vi "Subvi_Online_SVM_SWLDA_1세부통합.vi"(0 "rate":dbl=500.0 caption="Rate" format="%0.2f", 1 "Value":T1, 2 "Matrix":T1, 3 "in":T1, 5 "samples per channel":i32=25, 9 "Brain_data_source":dbl[][](array[numeric]) caption="EEG_Raw_Data" format="%0.3f", 11 "Target_Flash_Order":i64[][](array[numeric])) -> (4 "output-0~8":i32, 6 "decision":dbl[](array[numeric]), 8 "ERP_발생여부":bool, 10 "SWLDA":dbl[](array[numeric]), 13 "EPR_발생_total":i16[](array[numeric]), 14 "ERP_all":dbl[][](array[numeric]), 15 "ERP_Parameters":dbl[][](array[numeric]))   [LabVIEW 2014]
uses:
  <vilib>/Analysis/Matrix/Datatypes/RealMatrix.ctl
  <vilib>/Analysis/3filter.llb/Filter Passband Type.ctl
  <vilib>/Analysis/baseanly.llb/Mean (DBL).vi
  <vilib>/Analysis/3filter.llb/Butterworth Filter (DBL).vi
  <vilib>/Utility/file.llb/Read From Spreadsheet File (DBL).vi
  <vilib>/Analysis/Matrix/Numeric/Conversions/Array To Matrix - RA.vi
  <vilib>/Analysis/Matrix/Numeric/Multiply/Multiply - RM,RM.vi
  <vilib>/Analysis/Matrix/Numeric/Subtract/Subtract - RM,RM.vi
  <vilib>/Analysis/Matrix/Numeric/Conversions/Matrix To Array - RM.vi
  <vilib>/Analysis/NI_AALBase.lvlib
  <vilib>/Analysis/Matrix/NI_Matrix.lvlib
panel:
  # "Input Values"
  # "Output Values"
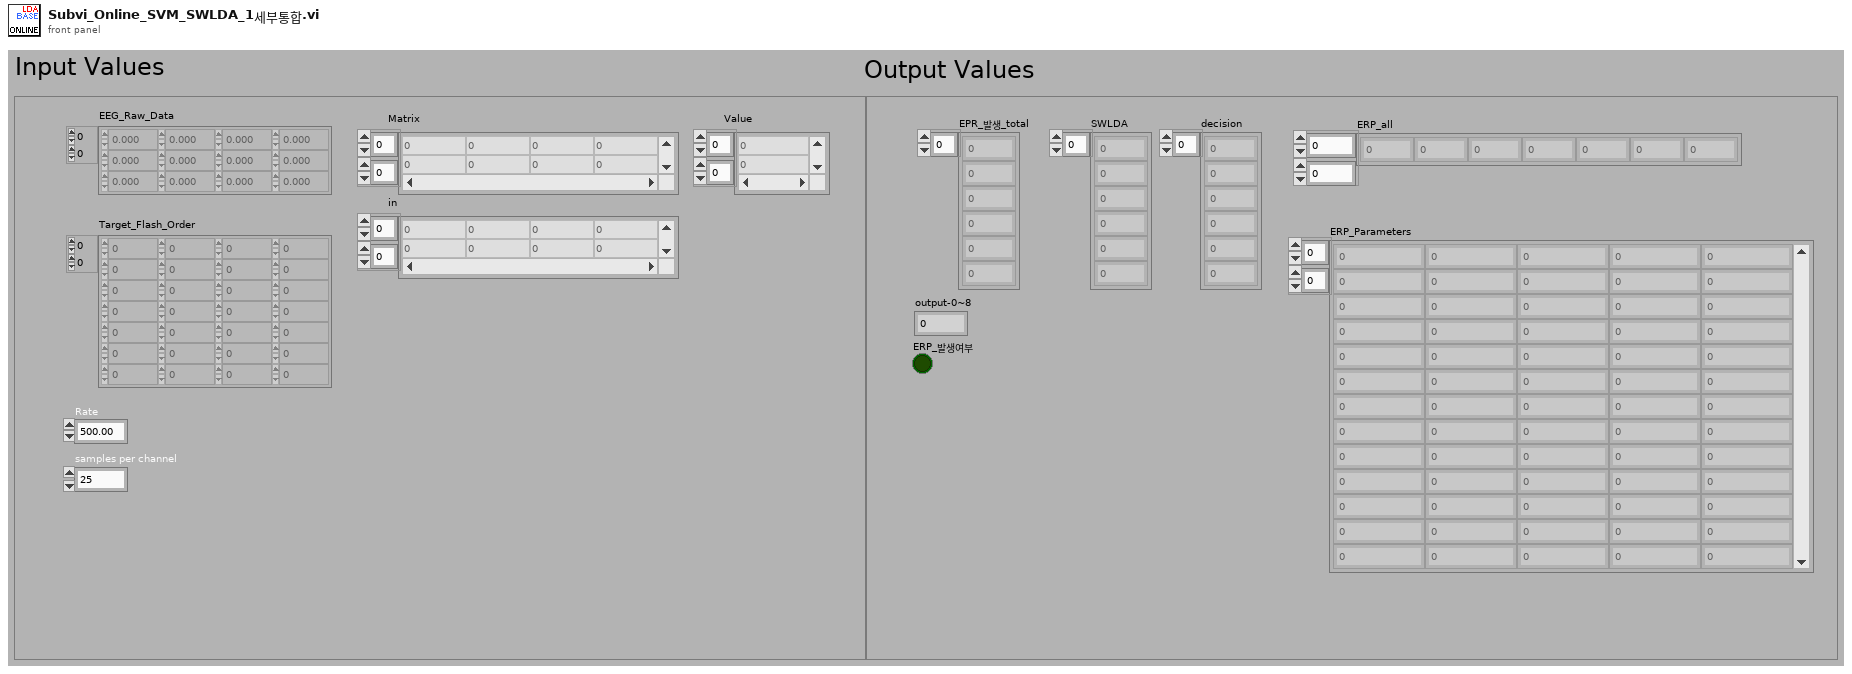
[diagram p1: front panel]
types:
  T1 = typedef "NI_Matrix.lvlib/RealMatrix.ctl" = dbl[][]
  T2 = typedef "NI_AALBase.lvlib/Filter Passband Type.ctl" = enum32{"Lowpass", "Highpass", "Bandpass", "Bandstop"}
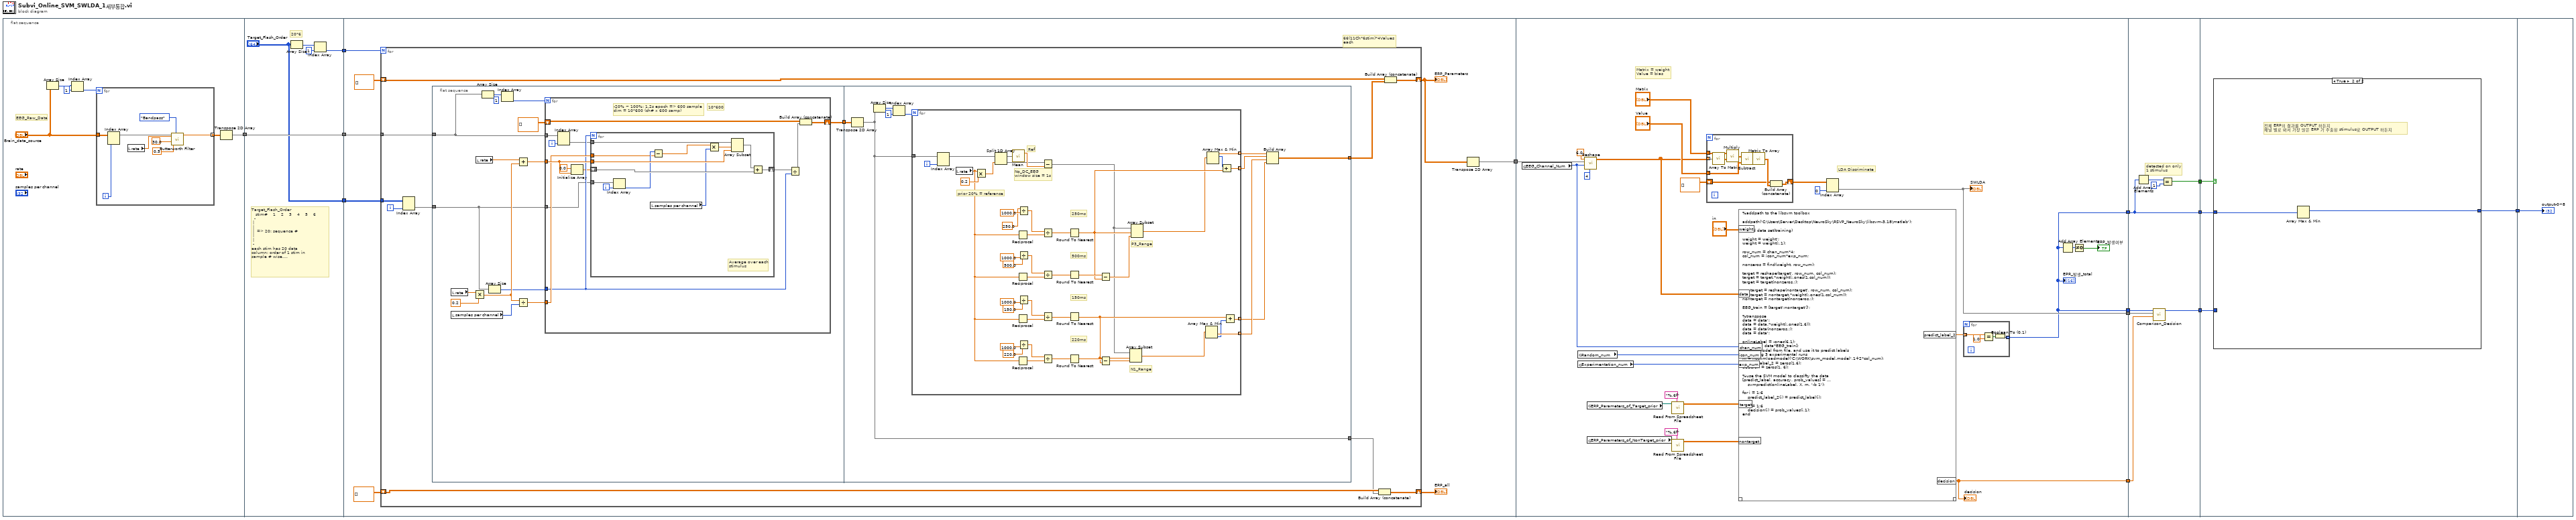
[diagram p0: block diagram]
diagram:
  n1 = flat-sequence {
    tunnel: [w14] -> w13
    tunnel: [w32] -> w12
    tunnel: ["Target_Flash_Order"] -> w11
    tunnel: w13 -> [w32]
    tunnel: [w29] -> w10
    tunnel: w12 -> [w40]
    tunnel: w11 -> [w39]
    tunnel: w10 -> [w38]
    tunnel: [w35] -> w9
    tunnel: w9 -> [w156]
    tunnel: [w150] -> w8
    tunnel: [w150] -> w7
    tunnel: [w164] -> w5
    tunnel: [w151] -> w2
    tunnel: [w190] -> w4
    tunnel: [w189] -> w3
    tunnel: [w188] -> w1
    tunnel: w2 -> [w183]
    tunnel: w5 -> [w184]
    tunnel: w7 -> [w185]
    tunnel: w8 -> [w190]
    tunnel: [w194] -> w6
    tunnel: w4 -> [w192]
    tunnel: w3 -> [w193]
    tunnel: w1 -> [w191]
    tunnel: w6 -> [w198]
    frame #0 {
      # "EEG_Raw_Data"
      n2 = Array Size(array="Brain_data_source") -> (size(s)=w18:i32[])
      n3 = Index Array(array=w18, index=1) -> (element=w16:i32)
      n4 = for {
        N: w16 -> [_]
        tunnel: "Brain_data_source" -> [w23]
        tunnel: [w22] -> w19 mode=indexing
        i -> [w20]
        n5 = Index Array(array=w23, index (col)=w20) -> (element=w21:dbl[])  [unwired: 1 in]
        n6 = local read "rate"() -> (w24:dbl)
        n7 = call-poly <vilib>:"Butterworth Filter.vi"("filter type"=Filter_Passband_Type."Bandpass", "low cutoff freq: fl"=0.5, "high cutoff freq: fh"=30.0, "sampling freq: fs"=w24, "X"=w21) -> ("Filtered X"=w22:dbl[])  [unwired: 3 in, 1 out]
      }
      n8 = Transpose 2D Array(2D array=w19) -> (transposed array=w14:dbl[][])
    }
    frame #1 {
      # "Target_Flash_Order\n   stim#    1    2    3    4    5    6    \n  -\n |\n |\n |  => 20: sequence # \n |\n |\n -\neach stim has 20 data\ncolumn: order of 1 stim in \nsample # wise...."
      # "20*6"
      n9 = Array Size(array="Target_Flash_Order") -> (size(s)=w31:i32[])
      n10 = Index Array(array=w31, index=1 ("인덱스")) -> (element=w29:i32)
    }
    frame #2 {
      # "66(11Ch*6stim)*4Values\neach"
      n11 = for {
        N: w38 -> [_]
        tunnel: w40 -> [w50]
        tunnel: w39 -> [w49]
        shift-right: [w46] -> w36
        shift-left: dbl[][] [] -> [w45]
        shift-right: [w43] -> w33
        shift-left: dbl[][] [] -> [w42]
        i -> [w48]
        n12 = Index Array(array=w49, index (col)=w48) -> (element=w47:i64[])  [unwired: 1 in]
        n13 = flat-sequence {
          tunnel: w50 -> [w53]
          tunnel: w47 -> [w57]
          tunnel: [w56] -> w51
          tunnel: w51 -> [w96]
          tunnel: [w95] -> w44
          tunnel: [w91] -> w41
          frame #0 {
            (unwired) 1 ("index")
            n14 = local read "rate"() -> (w61:dbl)
            n15 = local read "samples per channel"() -> (w59:i32)
            n16 = Multiply(x=w61, y=0.2) -> (x*y=w65:dbl)
            n17 = local read "rate"() -> (w63:dbl)
            n18 = Array Size(array=w53) -> (size(s)=w55:i32[])
            n19 = Array Size(array=w57) -> (size(s)=w58:i32)
            n20 = Index Array(array=w55) -> (element=w54:i32)  [unwired: 1 in]
            n21 = Add(x=w63, y=w65) -> (x+y=w64:dbl)
            n22 = Divide(x=w65, y=w59) -> (x/y=w62:dbl)
            n23 = for {
              N: w54 -> [_]
              tunnel: w64 -> [w78]
              tunnel: w62 -> [w77]
              tunnel: w58 -> [w76]
              tunnel: w53 -> [w75]
              tunnel: w57 -> [w74]
              shift-right: [w69] -> w56
              shift-left: dbl[][] [] -> [w68]
              i -> [w67]
              # "-20% ~ 100%: 1.2s epoch => 600 sample\ndim = 10*600 (ch# x 600 samp)"
              # "10*600"
              n24 = Index Array(array=w75, index (col)=w67) -> (element=w66:dbl[])  [unwired: 1 in]
              n25 = Initialize Array(0.0 ("element"), w78) -> (w73:dbl[])
              n26 = for {
                N: w76 -> [_]
                tunnel: w66 -> [w90]
                shift-right: [w87] -> w71
                shift-left: w73 -> [w88]
                tunnel: w78 -> [w86]
                tunnel: w74 -> [w84]
                tunnel: w77 -> [w82]
                i -> [w85]
                # "Average over each\nstimulus"
                n27 = Index Array(array=w84, index=w85) -> (element=w83:i64)
                n28 = local read "samples per channel"() -> (w79:i32)
                n29 = Subtract(x=w83, y=w82) -> (x-y=w80:dbl)
                n30 = Multiply(x=w80, y=w79) -> (x*y=w81:dbl)
                n31 = Array Subset(array=w90, index=w81, length=w86) -> (w89:dbl[])
                n32 = Add(x=w89, y=w88) -> (x+y=w87:dbl[])
              }
              n33 = Divide(x=w71, y=w76) -> (x/y=w70:dbl[])
              n34 = Build Array (concatenate)(w68, w70) -> (w69:dbl[][])
            }
          }
          frame #1 {
            n35 = Transpose 2D Array(2D array=w96) -> (transposed array=w91:dbl[][])
            n36 = Array Size(array=w91) -> (size(s)=w94:i32[])
            n37 = Index Array(array=w94, index=1) -> (element=w92:i32)
            n38 = for {
              N: w92 -> [_]
              tunnel: [w144] -> w100 mode=indexing
              tunnel: [w143] -> w99 mode=indexing
              tunnel: [w142] -> w98 mode=indexing
              tunnel: [w141] -> w97 mode=indexing
              tunnel: w91 -> [w103]
              i -> [w101]
              # "P3_Range"
              # "N1_Range"
              # "220ms"
              # "150ms"
              # "500ms"
              # "250ms"
              # "No_DC_EEG\nwindow size = 1s"
              # "Ref"
              # "prior 20% = reference"
              n39 = Index Array(array=w103, index (col)=w101) -> (element=w102:dbl[])  [unwired: 1 in]
              n40 = local read "rate"() -> (w117:dbl)
              n41 = Multiply(x=w117, y=0.2) -> (x*y=w139:dbl)
              n42 = Split 1D Array(array=w102, index=w139) -> (first subarray=w138:dbl[], second subarray=w134:dbl[])
              n43 = call-poly <vilib>:"Mean.vi"("X"=w138) -> ("mean"=w137:dbl)  [unwired: 1 out]
              n44 = Reciprocal(x=w117) -> (1/x=w133:dbl)
              n45 = Reciprocal(x=w117) -> (1/x=w132:dbl)
              n46 = Reciprocal(x=w117) -> (1/x=w131:dbl)
              n47 = Reciprocal(x=w117) -> (1/x=w130:dbl)
              n48 = Divide(x=250.0, y=1000.0) -> (x/y=w129:dbl)
              n49 = Divide(x=500.0, y=1000.0) -> (x/y=w128:dbl)
              n50 = Divide(x=150.0, y=1000.0) -> (x/y=w127:dbl)
              n51 = Divide(x=220.0, y=1000.0) -> (x/y=w126:dbl)
              n52 = Subtract(x=w134, y=w137) -> (x-y=w104:dbl[])
              n53 = Divide(x=w129, y=w133) -> (x/y=w116:dbl)
              n54 = Divide(x=w128, y=w132) -> (x/y=w115:dbl)
              n55 = Divide(x=w127, y=w131) -> (x/y=w114:dbl)
              n56 = Divide(x=w126, y=w130) -> (x/y=w113:dbl)
              n57 = Round To Nearest(number=w116) -> (nearest integer value=w107:dbl)
              n58 = Round To Nearest(number=w115) -> (nearest integer value=w112:dbl)
              n59 = Round To Nearest(number=w114) -> (nearest integer value=w109:dbl)
              n60 = Round To Nearest(number=w113) -> (nearest integer value=w111:dbl)
              n61 = Subtract(x=w112, y=w107) -> (x-y=w108:dbl)
              n62 = Subtract(x=w111, y=w109) -> (x-y=w110:dbl)
              n63 = Array Subset(array=w104, index=w109, length=w110) -> (w105:dbl[])
              n64 = Array Subset(array=w104, index=w107, length=w108) -> (w106:dbl[])
              n65 = Array Max & Min(array=w105) -> (min value=w142:dbl, min index (indices)=w135:i32)  [unwired: 2 out]
              n66 = Array Max & Min(array=w106) -> (max value=w144:dbl, max index (indices)=w136:i32)  [unwired: 2 out]
              n67 = Add(x=w136, y=w107) -> (x+y=w143:dbl)
              n68 = Add(x=w109, y=w135) -> (x+y=w141:dbl)
            }
            n69 = Build Array(w100, w99, w98, w97) -> (w95:dbl[][])
          }
        }
        n70 = Build Array (concatenate)(w42, w41) -> (w43:dbl[][])
        n71 = Build Array (concatenate)(w45, w44) -> (w46:dbl[][])
      }
      "ERP_Parameters" <- w36
      "ERP_all" <- w33
      n72 = Transpose 2D Array(2D array=w36) -> (transposed array=w35:dbl[][])
    }
    frame #3 {
      # "Matrix = weight\nValue = bias"
      # "LDA Discriminate"
      n73 = global read "Control_Panel_정리.vi" "EEG_Channel_Num"() -> (w147:i32)
      n74 = global read "Control_Panel_정리.vi" "Random_num"() -> (w146:i32)
      n75 = global read "Control_Panel_정리.vi" "Experimentation_num"() -> (w145:i32)
      n76 = call "Reshape.vi"("Numeric"=4, "EEG_Channel_Num"=w147, "all rows"=w156, "Numeric 2"=6.0) -> ("Array"=w153:dbl[][])  [unwired: 7 in]
      n77 = global read "Control_Panel_정리.vi" "ERP_Parameters_of_Target_prior"() -> (w162:path)
      n78 = global read "Control_Panel_정리.vi" "ERP_Parameters_of_NonTarget_prior"() -> (w160:path)
      n79 = call-poly <vilib>:"Read From Spreadsheet File.vi"("format (%.3f)"="%.6f", "file path (dialog if empty)"=w162) -> ("all rows"=w159:dbl[][])  [unwired: 5 in, 4 out]
      n80 = call-poly <vilib>:"Read From Spreadsheet File.vi"("format (%.3f)"="%.6f", "file path (dialog if empty)"=w160) -> ("all rows"=w158:dbl[][])  [unwired: 5 in, 4 out]
      n81 = for {
        tunnel: "Matrix" -> [w174]
        tunnel: "Value" -> [w180]
        shift-right: [w177] -> w167
        shift-left: dbl[][] [] -> [w176]
        tunnel: w153 -> [w175] mode=indexing
        n82 = call-poly <vilib>:"Array To Matrix.vi"("Real 1D Array"=w175) -> ("Real Matrix (Column Vector)"=w179:T1)
        n83 = call-poly <vilib>:"Multiply.vi"("Real Matrix B"=w179, "Real Matrix A"=w174) -> ("A * B"=w182:T1)
        n84 = call-poly <vilib>:"Subtract.vi"("Real Matrix B"=w180, "Real Matrix A"=w182) -> ("A - B"=w181:T1)
        n85 = call-poly <vilib>:"Matrix To Array.vi"("Real Matrix"=w181) -> ("Real 2D Array"=w178:dbl[][])
        n86 = Build Array (concatenate)(w176, w178) -> (w177:dbl[][])
      }
      n87 = script code="%addpath to the libsvm toolbox\n\naddpath('C:\\Users\\Server\\Desktop\\NeuroSky\\RSVP_NeuroSky\\libsvm-3.18\\matlab');\n\n%read data set(training)\n\nweight = weight';\nweight = weight(:,1);\n\nrow_num = chan_num*4;\ncol_num = icon_num*exp_num;\n\nnonzeros = find(weight, row_num);\n\ntarget = reshape(target', row_num, col_num);\ntarget = target.*weight(:,ones(1,col_num));\ntarget = target(nonzeros,:);\n\nnontarget = reshape(nontarget', row_num, col_num);\nnontarget = nontarget.*weight(:,ones(1,col_num));\nnontarget = nontarget(nonzeros,:);\n\nEEG_train = [target';nontarget']';\n\n%transpose\ndata = data';\ndata = data.*weight(:,ones(1,6));\ndata = data(nonzeros,:);\ndata = data';\n\nonlineLabel = -ones(6,1);\nX = [(1:6)' data*EEG_train];\n% load model from file, and use it to predict labels\n% training 3 experimental runs\nm = libsvmloadmodel('C:\\WORK\\svm_model.model',1+2*col_num);\npredict_label_2 = zeros(1,6);\ndecision = zeros(1, 6);\n\n%use the SVM model to classifty the data\n[predict_label, accuracy, prob_values] = ...\n    svmpredict(onlineLabel, X, m, '-b 1');\n\nfor i = 1:6\n    predict_label_2(i) = predict_label(i);\nend\nfor i = 1:6\n    decision(i) = prob_values(i,1);\nend"("weight"="in", "target"=w159, "nontarget"=w158, "data"=w153, "chan_num"=w147, "icon_num"=w146, "exp_num"=w145) -> ("predict_label_2"=w157:dbl[], "decision"=w151:dbl[])  [unwired: 1 in, 1 out]
      "decision" <- w151
      n88 = Index Array(array=w167, index (col)=0 ("비활성화된 인덱스 (열)")) -> (element=w164:dbl[])  [unwired: 1 in]
      "SWLDA" <- w164
      n89 = for {
        tunnel: w157 -> [w173] mode=indexing
        tunnel: [w172] -> w150 mode=indexing
        n90 = Equal?(x=w173, y=1.0) -> (x = y?=w170:bool)
        n91 = Boolean To (0,1)(Boolean=w170) -> (0, 1=w172:i16)
      }
      "EPR_발생_total" <- w150
      n92 = Add Array Elements(numeric array=w150) -> (sum=w149:i16)
      n93 = Not Equal To 0?(x=w149) -> (x != 0?=→"ERP_발생여부":bool)
    }
    frame #4 {
      # "detected on only\n1 stimulus"
      n94 = Add Array Elements(numeric array=w190) -> (sum=w187:i16)
      n95 = call "Comparison_Decision.vi"("decision"=w183, "SWLDA"=w184, "EPR_발생_total"=w185) -> ("selected"=w188:i32)  [unwired: 8 in]
      n96 = Equal?(x=w187, y=i16 1) -> (x = y?=w189:bool)
    }
    frame #5 {
      n97 = case shown="True" w193 {
        tunnel: [w195 w197] -> w194
        tunnel: w192 -> [_ w196]
        tunnel: w191 -> [w195 _]
        frame False {
        }
        frame True {
          # "전체 ERP의 결과를 OUTPUT 하든지\n채널 별로 봐서 가장 많은 ERP 가 추출된 stimulus로 OUTPUT 하든지"
          n98 = Array Max & Min(array=w196) -> (max index (indices)=w197:i32)  [unwired: 3 out]
        }
      }
    }
    frame #6 {
      "output-0~8" <- w198
    }
  }
